vi "Recovery SN.vi"(8 "error in (no error)":errorcluster caption="entrée d'erreur (pas d'erreur)", 11 "Firebase Benches en entrée":refnum<class "Firebase Recovery_SN.lvclass">) -> (0 "error out":errorcluster caption="sortie d'erreur", 3 "Firebase Benches en sortie":refnum<class "Firebase Recovery_SN.lvclass">)   [LabVIEW 2020, in "Library Instrument & Equipement.lvlib" / "Library FireBase.lvlib" / "Firebase Recovery_SN.lvclass"]
doc: "Returns data according to Value_To_Find on Collection_to_find Use Nb_To_Read to determine the number to read\nPlease initialise the following values before use the VI\n - Name BDD\n - Value to find\n - API Key\n - Field Filter\n - Field Order\n - Collection_to_find\n\nIf there is no Field order -> Field Order=Field Filter"
uses:
  Firebase Recovery_SN.lvclass
  C:/Users/ngarcin/OneDrive - Altyor/Standard TB/Class/Firebase/Source/Firebase Driver/Firebase Driver.lvclass
  Firebase Recovery_SN.lvclass/Firebase Recovery_SN.ctl
  JSON API/JSON Value/Set from JSON string.vi
  JSON API/JSON Value/JSON Value.lvclass
  JSON API/Variant JSON/Variant JSON.lvlib
  JSON API/Get Polymorphic/JSON GetSet.lvlib
  Firebase Driver/Firebase Driver.lvclass
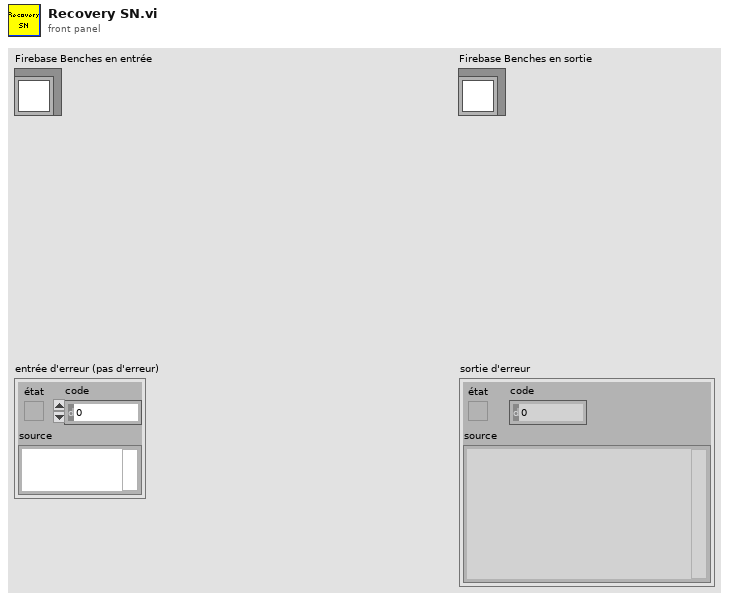
[diagram p1: front panel]
types:
  T1 = cluster{"name":string, "fields":cluster{"Value":cluster{"stringValue":string}}}[]
  T2 = cluster{"documents":cluster{"name":string, "fields":cluster{"Value":cluster{"stringValue":string}}}[]}
  T3 = cluster{"name":string, "fields":cluster{"Value":cluster{"stringValue":string}}}
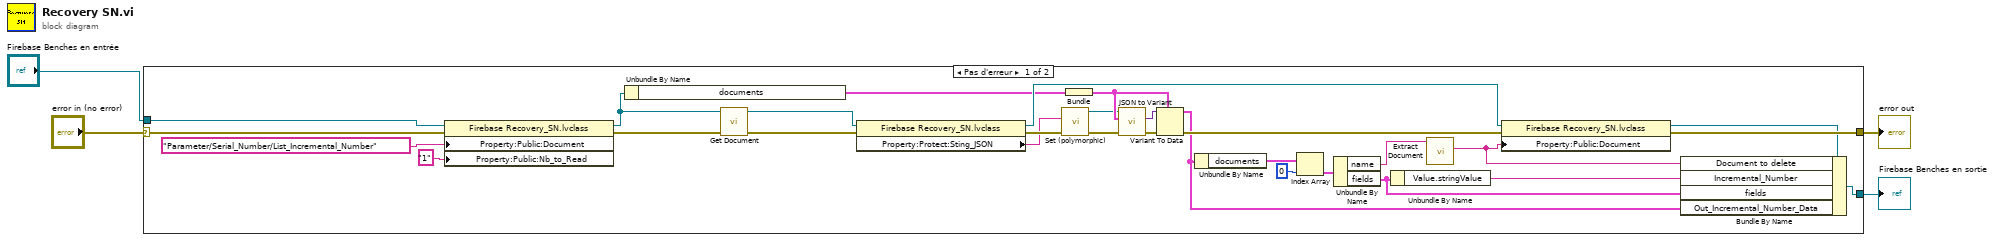
[diagram p0: block diagram]
diagram:
  n1 = case shown="Pas d'erreur" "error in (no error)" {
    selector: "error in (no error)" -> [w32 w35]
    tunnel: "Firebase Benches en entrée" -> [w33 w34]
    tunnel: [w30 w35] -> w3
    tunnel: [w31 w34] -> w2
    frame No Error {
      n2 = property class="Firebase Recovery_SN.lvclass"(reference=w33, error in=w32, "Property:Public:Document"="Parameter/Serial_Number/List_Incremental_Number" ("Collection_to_find"), "Property:Public:Nb_to_Read"="1" ("Nb_to_Read")) -> (reference out=w8:refnum<class "Firebase Recovery_SN.lvclass">, error out=w28:errorcluster)
      n3 = Unbundle By Name(w8) -> ("documents"=w20:T1)
      n4 = call-dynamic "Get Document.vi"("error in (no error)"=w28, "Firebase (Default) en entrée"=w8) -> ("error out"=w12:errorcluster, "Firebase (Default) en sortie"=w11:refnum<class "Firebase Recovery_SN.lvclass">)  [unwired: 8 in]
      n5 = property class="Firebase Recovery_SN.lvclass"(reference=w11, error in=w12) -> (reference out=w25:refnum<class "Firebase Recovery_SN.lvclass">, error out=w18:errorcluster, "Property:Protect:Sting_JSON"=w17:string)
      n6 = call-poly "Set (polymorphic).vi"("error in (no error)"=w18, "JSON stream"=w17) -> ("error out"=w16:errorcluster, "JSON Value out"=w14:refnum<class "JSON Value.lvclass">)  [unwired: 7 in, 1 out]
      n7 = Bundle("documents"=w20) -> (w21:T2)  [unwired: 1 in]
      n8 = call "JSON to Variant.vi"("error in (no error)"=w16, "Variant (Data Type)"=w21, "JSON Value"=w14) -> ("error out"=w15:errorcluster, "Variant out"=w19:variant)  [unwired: 7 in]
      n9 = Variant To Data(error in=w15, type=w21, Variant=w19) -> (data=w9:T2, error out=w22:errorcluster)
      n10 = Unbundle By Name(w9) -> ("documents"=w23:T1)
      n11 = Index Array(array=w23, index=0 ("indice")) -> (element=w24:T3)
      n12 = Unbundle By Name(w24) -> ("name"=w26:string, "fields"=w7:cluster{"Value":cluster{"stringValue":string}})
      n13 = Unbundle By Name(w7) -> ("Value.stringValue"=w6:string)
      n14 = call "Extract Document.vi"("Name"=w26) -> ("Source"=w5:string)  [unwired: 9 in, 1 out]
      n15 = property class="Firebase Recovery_SN.lvclass"(reference=w25, error in=w22, "Property:Public:Document"=w5) -> (reference out=w10:refnum<class "Firebase Recovery_SN.lvclass">, error out=w30:errorcluster)
      n16 = Bundle By Name(cluster=w10, "Document to delete"=w5, "Incremental_Number"=w6, "fields"=w7, "Out_Incremental_Number_Data"=w9) -> (w31:refnum<class "Firebase Recovery_SN.lvclass">)
    }
    frame Error {
    }
  }
  "error out" <- w3
  "Firebase Benches en sortie" <- w2
